vi "read from serial.vi"(8 "error in (no error)":errorcluster, 11 "SIM_Roda_Filtros in":refnum<class "SIM_Roda_Filtros.lvclass">) -> (0 "error out":errorcluster, 3 "SIM_Roda_Filtros out":refnum<class "SIM_Roda_Filtros.lvclass">)   [LabVIEW 2018, in "SIM_Roda_Filtros.lvclass"]
uses:
  SIM_Roda_Filtros.lvclass
  C:/Users/Denis/Desktop/FWCS/FWCS/Roda_Filtros/Roda_Filtros.lvclass
  Roda_Filtros/Roda_Filtros.lvclass/Roda_Filtros.ctl
  Roda_Filtros/Roda_Filtros.lvclass
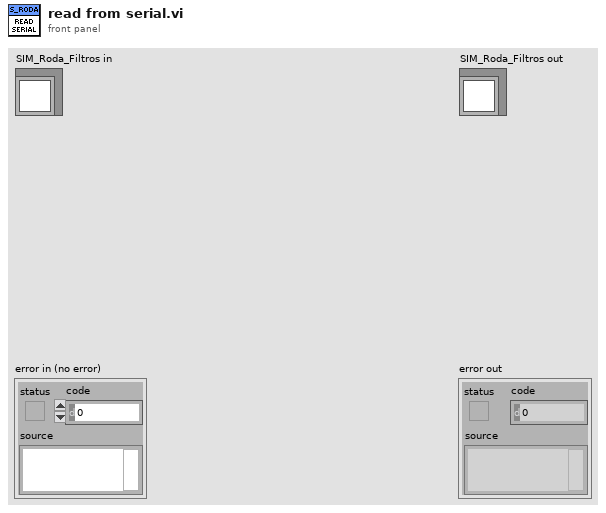
[diagram p1: front panel]
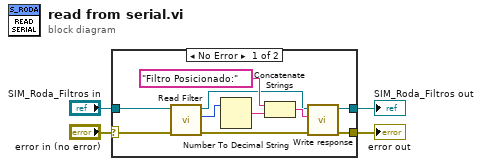
[diagram p0: block diagram]
diagram:
  n1 = case shown="No Error" "error in (no error)" {
    selector: "error in (no error)" -> [w13 w15]
    tunnel: "SIM_Roda_Filtros in" -> [w14 w16]
    tunnel: [w12 w16] -> w2
    tunnel: [w11 w15] -> w1
    frame No Error {
      n2 = call "Read Filter.vi"("error in (no error)"=w13, "Roda_Filtros in"=w14) -> ("error out"=w7:errorcluster, "Filter"=w6:u16, "Roda_Filtros out"=w8:refnum<class "SIM_Roda_Filtros.lvclass">)  [unwired: 7 in]
      n3 = Number To Decimal String(number=w6) -> (decimal integer string=w5:string)  [unwired: 1 in]
      n4 = Concatenate Strings("Filtro Posicionado:", w5) -> (w9:string)
      n5 = call-dynamic "Write response.vi"("error in (no error)"=w7, "response"=w9, "Roda_Filtros in"=w8) -> ("error out"=w11:errorcluster, "Roda_Filtros out"=w12:refnum<class "SIM_Roda_Filtros.lvclass">)  [unwired: 7 in]
    }
    frame Error {
    }
  }
  "error out" <- w1
  "SIM_Roda_Filtros out" <- w2
